vi "Ler_encoder_modificado.vi"() -> (0 "error out":errorcluster, 3 "Posição":i32)   [LabVIEW 2018]
uses:
  <vilib>/DAQmx/write.llb/DAQmx Write (Digital Bool 1Line 1Point).vi
  <vilib>/DAQmx/read.llb/DAQmx Read (Analog 1D DBL 1Chan NSamp).vi
  <vilib>/DAQmx/create/channels.llb/DAQmx Create Channel (DO-Digital Output).vi
  <vilib>/DAQmx/miscellaneous.llb/DAQmx Fill In Error Info.vi
  <vilib>/DAQmx/create/channels.llb/DAQmx Create Channel (CO-Pulse Generation-Frequency).vi
  <vilib>/DAQmx/configure/timing.llb/DAQmx Timing (Implicit).vi
  <vilib>/DAQmx/configure/trigger.llb/DAQmx Start Trigger (Digital Edge).vi
  <vilib>/DAQmx/create/channels.llb/DAQmx Create Channel (AI-Voltage-Basic).vi
  <vilib>/DAQmx/configure/timing.llb/DAQmx Timing (Sample Clock).vi
panel:
  out "Waveform Chart 2":dbl(graph)
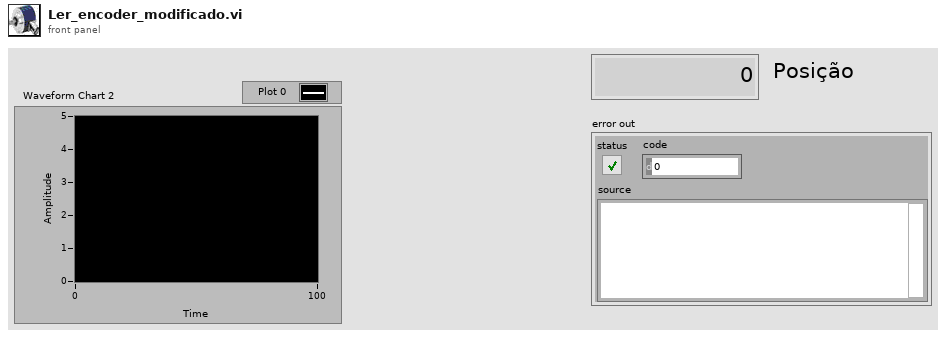
[diagram p1: front panel]
types:
  T1 = cluster{"Acionador":tag, "Clock":tag, "Canal Analogico":tag, "Trigger":tag}
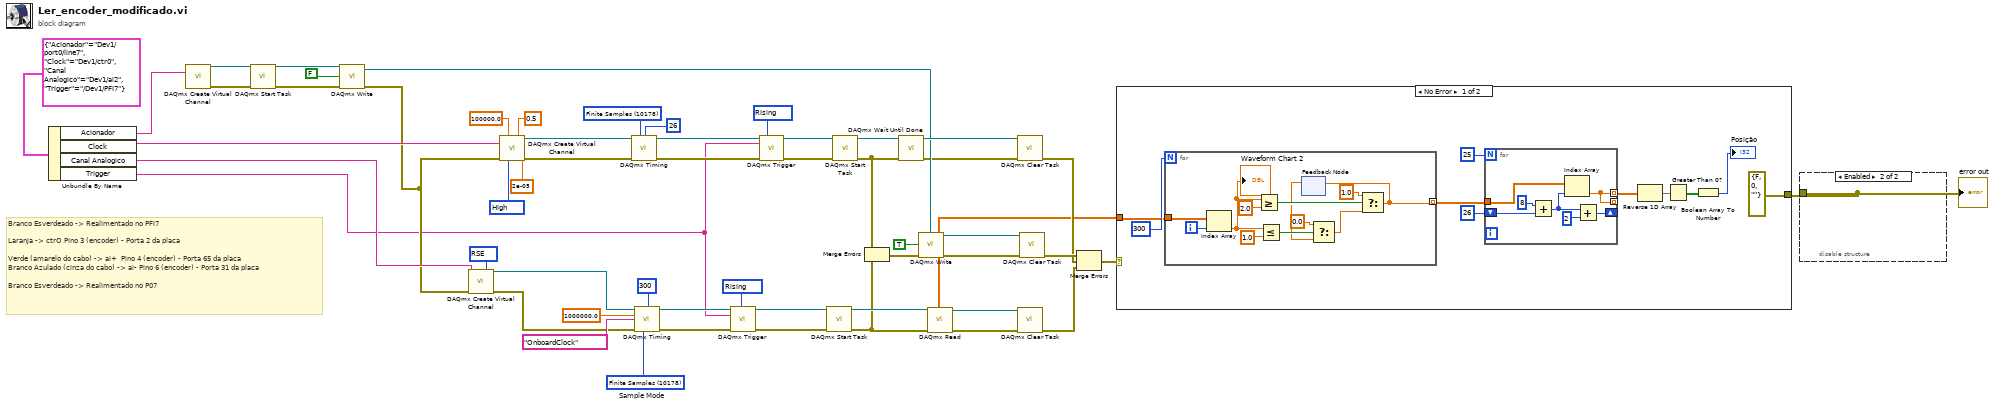
[diagram p0: block diagram]
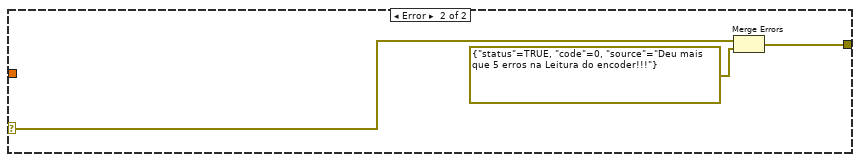
[diagram p2: hidden frame]
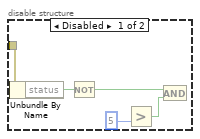
[diagram p3: hidden frame]
diagram:
  w12 = 10083 items=["default"=-1, "RSE"=10083, "NRSE"=10078, "Differential"=10106, "Pseudodifferential"=12529] ("Terminal Configuration")
  w16 = 10280 items=["Rising"=10280, "Falling"=10171] ("Edge")
  w6 = 10178 items=["Finite Samples"=10178, "Continuous Samples"=10123, "Hardware Timed Single Point"=12522]  # Sample Mode
  w32 = 10280 items=["Rising"=10280, "Falling"=10171] ("edge")
  w31 = 10192 items=["High"=10192, "Low"=10214] ("idle state")
  w24 = 10178 items=["Finite Samples"=10178, "Continuous Samples"=10123] ("sample mode")
  # "Branco Esverdeado -> Realimentado no PFI7\n\nLaranja -> ctrO Pino 3 (encoder) - Porta 2 da placa\n\nVerde (amarelo do cabo) -> ai+  Pino 4 (encoder) - Porta 65 da placa\nBranco Azulado (cinza do cabo) -> ai- Pino 6 (encoder) - Porta 31 da placa\n\nBranco Esverdeado -> Realimentado no P07"
  n1 = Unbundle By Name(T1 {"Acionador"="Dev1/port0/line7", "Clock"="Dev1/ctr0", "Canal Analogico"="Dev1/ai2", "Trigger"="/Dev1/PFI7"} ("Portas")) -> ("Acionador"=w51:tag, "Clock"=w50:tag, "Canal Analogico"=w49:tag, "Trigger"=w1:tag)
  n2 = call-poly <vilib>:"DAQmx Create Virtual Channel.vi"("lines"=w51) -> ("task out"=w53:refnum<k21>, "error out"=w54:errorcluster)  [unwired: 13 in]
  n3 = call <vilib>:"DAQmx Start Task.vi"("task/channels in"=w53, "error in"=w54) -> ("task out"=w39:refnum<k21>, "error out"=w38:errorcluster)  [unwired: 12 in]
  n4 = call-poly <vilib>:"DAQmx Write.vi"("task/channels in"=w39, "data"=FALSE, "error in"=w38) -> ("task out"=w35:refnum<k21>, "error out"=w33:errorcluster)  [unwired: 10 in, 1 out]
  n5 = call-poly <vilib>:"DAQmx Create Virtual Channel.vi"("input terminal configuration"=w12, "physical channels"=w49, "error in"=w33) -> ("task out"=w8:refnum<k21>, "error out"=w7:errorcluster)  [unwired: 11 in]
  n6 = call-poly <vilib>:"DAQmx Create Virtual Channel.vi"("frequency"=100000.0, "duty cycle"=0.5, "counter"=w50, "error in"=w33, "idle state"=w31, "initial delay"=2e-05) -> ("task out"=w23:refnum<k21>, "error out"=w22:errorcluster)  [unwired: 8 in]
  n7 = call-poly <vilib>:"DAQmx Timing.vi"("task/channels in"=w23, "sample mode"=w24, "samples per channel"=26, "error in"=w22) -> ("task out"=w25:refnum<k21>, "error out"=w26:errorcluster)  [unwired: 10 in]
  n8 = call-poly <vilib>:"DAQmx Timing.vi"("task/channels in"=w8, "sample mode"=w6, "samples per channel"=300 ("Number of Samples"), "rate"=1000000.0 ("Sample Rate"), "source"=tag "OnboardClock" ("Sample Clock Source"), "error in"=w7) -> ("task out"=w17:refnum<k21>, "error out"=w18:errorcluster)  [unwired: 8 in]
  n9 = call-poly <vilib>:"DAQmx Trigger.vi"("task/channels in"=w17, "source"=w1, "edge"=w16, "error in"=w18) -> ("task out"=w9:refnum<k21>, "error out"=w10:errorcluster)  [unwired: 10 in]
  n10 = call-poly <vilib>:"DAQmx Trigger.vi"("task/channels in"=w25, "source"=w1, "edge"=w32, "error in"=w26) -> ("task out"=w20:refnum<k21>, "error out"=w19:errorcluster)  [unwired: 10 in]
  n11 = call <vilib>:"DAQmx Start Task.vi"("task/channels in"=w9, "error in"=w10) -> ("task out"=w11:refnum<k21>, "error out"=w4:errorcluster)  [unwired: 12 in]
  n12 = call <vilib>:"DAQmx Start Task.vi"("task/channels in"=w20, "error in"=w19) -> ("task out"=w21:refnum<k21>, "error out"=w5:errorcluster)  [unwired: 12 in]
  n13 = Merge Errors(w5, w4) -> (w3:errorcluster)
  n14 = call <vilib>:"DAQmx Wait Until Done.vi"("task/channels in"=w21, "error in"=w5) -> ("task out"=w46:refnum<k21>, "error out"=w34:errorcluster)  [unwired: 12 in]
  n15 = call-poly <vilib>:"DAQmx Write.vi"("task/channels in"=w35, "data"=TRUE ("stop (T)"), "error in"=w3) -> ("task out"=w36:refnum<k21>, "error out"=w40:errorcluster)  [unwired: 10 in, 1 out]
  n16 = call-poly <vilib>:"DAQmx Read.vi"("task/channels in"=w11, "error in"=w4) -> ("task out"=w43:refnum<k21>, "data"=w41:dbl[], "error out"=w44:errorcluster)  [unwired: 11 in]
  n17 = call <vilib>:"DAQmx Clear Task.vi"("task in"=w46, "error in"=w34) -> ("error out"=w45:errorcluster)  [unwired: 13 in]
  n18 = call <vilib>:"DAQmx Clear Task.vi"("task in"=w43, "error in"=w44) -> ("error out"=w42:errorcluster)  [unwired: 13 in]
  n19 = call <vilib>:"DAQmx Clear Task.vi"("task in"=w36, "error in"=w40) -> ("error out"=w47:errorcluster)  [unwired: 13 in]
  n20 = Merge Errors(w47, w45, w42) -> (w48:errorcluster)
  n21 = case shown="No Error" w48 {
    selector: w48 -> [_ w87]
    tunnel: [errorcluster {"status"=FALSE, "code"=0, "source"=""} ("error IO") w86] -> w55
    tunnel: w41 -> [w57 _]
    frame No Error {
      n22 = for {
        N: 300 -> [_]
        tunnel: w57 -> [w84]
        tunnel: [w75] -> w62 mode=indexing
        i -> [w83]
        n23 = Index Array(array=w84, index=w83) -> (element=w73:dbl)
        "Waveform Chart 2" <- w73
        n24 = Greater Or Equal?(x=w73, y=2.0) -> (x >= y?=w82:bool)
        n25 = Less Or Equal?(x=w73, y=1.0) -> (x <= y?=w80:bool)
        n26 = feedback #1() -> (w74:dbl)  [unwired: 1 in]
        n27 = Select(t=0.0, s=w80, f=w74) -> (s? t:f=w79:dbl)
        n28 = Select(t=1.0, s=w82, f=w79) -> (s? t:f=w75:dbl)
        n29 = feedback-in #1(w75) -> ()
      }
      n30 = for {
        N: 25 -> [_]
        tunnel: w62 -> [w71]
        tunnel: [w66] -> w56 mode=indexing
        shift-right: [w69] -> _
        shift-left: 26 -> [w68]
        tunnel: [w66] -> _ mode=indexing
        n31 = Add(x=8, y=w68) -> (x+y=w67:i32)
        n32 = Index Array(array=w71, index=w67) -> (element=w66:dbl)
        n33 = Add(x=w67, y=2) -> (x+y=w69:i32)
      }
      n34 = Reverse 1D Array(array=w56) -> (reversed array=w60:dbl[])
      n35 = Greater Than 0?(x=w60) -> (x > 0?=w61:bool[])
      n36 = Boolean Array To Number(Boolean array=w61) -> (number=→"Posição":i32)
    }
    frame Error {
      n37 = Merge Errors(w87, errorcluster {"status"=TRUE, "code"=0, "source"="Deu mais que 5 erros na Leitura do encoder!!!"} ("error in")) -> (w86:errorcluster)
    }
  }
  "error out" <- w55
  n38 = disable-structure shown="Enabled" {
    disable-tunnel: w55 -> [w92 _]
    frame Disabled {
      n39 = Unbundle By Name(w92) -> ("status"=w91:bool)
      n40 = Not(x=w91) -> (.not. x?=w88:bool)
      n41 = Greater?(y=5) -> (0:w89:bool)  [unwired: 1 in]
      n42 = And(x=w88, y=w89) -> ()  [unwired: 1 out]
    }
    frame Enabled {
    }
  }
